vi "io_query_with_OPC_synchro.vi"(7 "Timeout in (0 = OPC timeout)":u32, 8 "error in":errorcluster, 9 "bytes to read (Read all available)":u32, 10 "write buffer":string, 11 "VISA resource name":refnum<visa-resource-name>) -> (0 "error out":errorcluster, 2 "read buffer":string, 3 "VISA resource name out":refnum<visa-resource-name>)   [LabVIEW 2014, in "rszvl_rsidr_core.lvlib"]
uses:
  rszvl_rsidr_core.lvlib
  type_Attribute.ctl
  type_Attribute_Data_Type.ctl
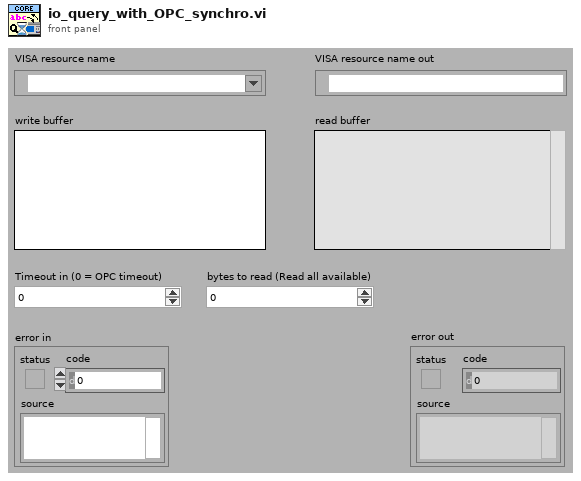
[diagram p1: front panel]
types:
  T1 = typedef "rszvl_rsidr_core.lvlib/type_Session_Data.ctl" = cluster{"Instr type":string, "Instr type for err. msg.":string, "Installed Options":string[], "OPC Timeout":i32, "Query Instrument Status":bool, "Check Range":bool, "Check Options":bool, "Add LF to Write":bool, "Simulate":bool, "Logging":bool, "Logging params":variant, "Interface Type":enum16{"Unknown", "GPIB", "VXI", "GPIB_VXI", "ASRL", "PXI", "TCPIP", "USB", "SOCKET"}, "Fast Sweep":i32, "AdditionalFlags":i32, "WaitBeforeWrite":i32, "WaitBeforeRead":i32, "BinDataChunkSize":i64}
  T2 = enum16{"Unknown", "GPIB", "VXI", "GPIB_VXI", "ASRL", "PXI", "TCPIP", "USB", "SOCKET"}
  T3 = typedef "rszvl_rsidr_core.lvlib/type_Attribute.ctl" = cluster{"Identifier":string, "Descriptive name":string, "Data Type":T4, "Command":string, "Access":u16, "Range Table":string, "Read Callback":string, "Write Callback":string, "Range Callback":string, "Check Callback":string, "Rngtable Callback":string, "Coerce Callback":string, "Supported Models":string, "Instrument Options":string, "Repeated Capabilities":string, "Check Status Callback":string, "Index":i32, "Flag: OPC Wait":bool, "Flag: Dont check status":bool, "Flag: Cache Only":bool}
  T4 = typedef "rszvl_rsidr_core.lvlib/type_Attribute_Data_Type.ctl" = enum16{"Integer 32", "Double", "String", "Boolean", "None", "Integer 64"}
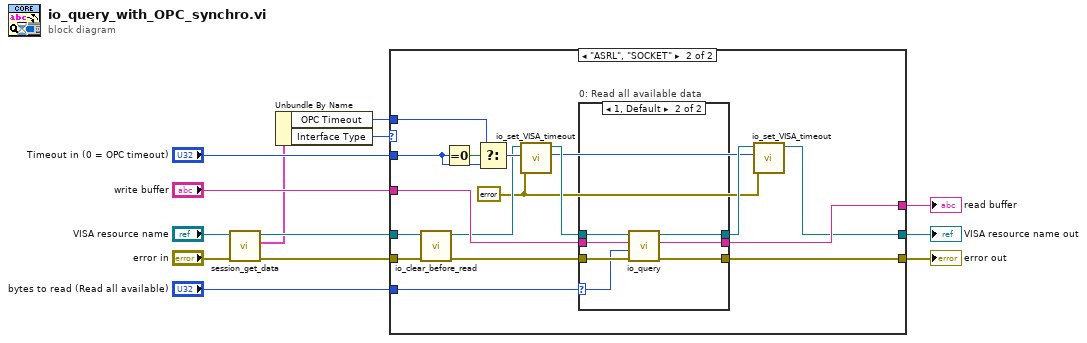
[diagram p0: block diagram]
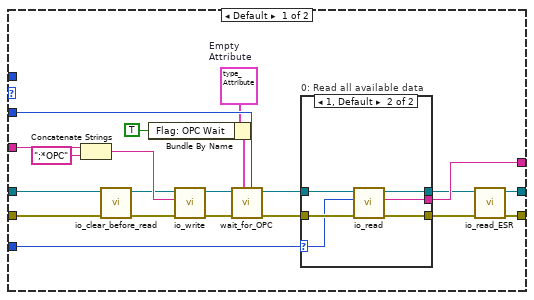
[diagram p2: hidden frame]
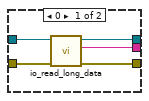
[diagram p3: hidden frame]
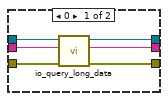
[diagram p4: hidden frame]
diagram:
  n1 = call "session_get_data.vi"("error in"="error in", "VISA resource name"="VISA resource name") -> ("error out"=w5:errorcluster, "Session User Data out"=w2:T1, "VISA resource name out"=w4:refnum<visa-resource-name>)  [unwired: 7 in]
  n2 = Unbundle By Name(w2) -> ("OPC Timeout"=w1:i32, "Interface Type"=w3:T2)
  n3 = case shown="\"ASRL\", \"SOCKET\"" w3 {
    tunnel: "Timeout in (0 = OPC timeout)" -> [w34 w53]
    tunnel: "write buffer" -> [w33 w57]
    tunnel: [w32 w62] -> w11
    tunnel: "bytes to read (Read all available)" -> [w31 w61]
    tunnel: [w30 w58] -> w9
    tunnel: [w29 w48] -> w8
    tunnel: w5 -> [w15 w60]
    tunnel: w4 -> [w14 w59]
    tunnel: w1 -> [_ w52]
    frame Default {
      w20 = T3 {"Identifier"="", "Descriptive name"="", "Data Type"=enum."Integer 32", "Command"="", "Access"=2, "Range Table"="", "Read Callback"="", "Write Callback"="", "Range Callback"="", "Check Callback"="", "Rngtable Callback"="", "Coerce Callback"="", "Supported Models"="", "Instrument Options"="", "Repeated Capabilities"="", "Check Status Callback"="", "Index"=0, "Flag: OPC Wait"=FALSE, "Flag: Dont check status"=FALSE, "Flag: Cache Only"=FALSE}  # Empty Attribute
      n4 = Concatenate Strings(w33, ";*OPC" ("string")) -> (w28:string)
      n5 = call "io_clear_before_read.vi"("error in"=w15, "VISA resource name"=w14) -> ("error out"=w26:errorcluster, "VISA resource name out"=w25:refnum<visa-resource-name>)  [unwired: 8 in]
      n6 = Bundle By Name(cluster=w20, "Flag: OPC Wait"=TRUE) -> (w19:T3)
      n7 = call "io_write.vi"("error in"=w26, "write buffer"=w28, "VISA resource name"=w25) -> ("error out"=w24:errorcluster, "VISA resource name out"=w23:refnum<visa-resource-name>)  [unwired: 7 in]
      n8 = call "wait_for_OPC.vi"("Timeout in (0 = OPC timeout)"=w34, "Attribute"=w19, "error in"=w24, "VISA resource name"=w23) -> ("error out"=w22:errorcluster, "VISA resource name out"=w21:refnum<visa-resource-name>)  [unwired: 6 in]
      n9 = case "0: Read all available data" shown="1, Default" w31 {
        selector: w31 -> [_ w41]
        tunnel: w22 -> [w39 w45]
        tunnel: w21 -> [w38 w44]
        tunnel: [w37 w43] -> w17
        tunnel: [w36 w42] -> w16
        tunnel: [w35 w40] -> w32
        frame 0 {
          n10 = call "io_read_long_data.vi"("error in"=w39, "VISA resource name"=w38) -> ("error out"=w37:errorcluster, "read buffer"=w35:string, "VISA resource name out"=w36:refnum<visa-resource-name>)  [unwired: 6 in, 1 out]
        }
        frame 1, Default {
          n11 = call "io_read.vi"("error in"=w45, "byte count (2048)"=w41, "VISA resource name"=w44) -> ("error out"=w43:errorcluster, "read buffer"=w40:string, "VISA resource name out"=w42:refnum<visa-resource-name>)  [unwired: 5 in, 1 out]
        }
      }
      n12 = call "io_read_ESR.vi"("error in"=w17, "VISA resource name"=w16) -> ("error out"=w30:errorcluster, "VISA resource name out"=w29:refnum<visa-resource-name>)  [unwired: 7 in, 1 out]
    }
    frame "ASRL", "SOCKET" {
      w47 = errorcluster {"status"=FALSE, "code"=0, "source"=""} ("error in")
      n13 = call "io_clear_before_read.vi"("error in"=w60, "VISA resource name"=w59) -> ("error out"=w56:errorcluster, "VISA resource name out"=w51:refnum<visa-resource-name>)  [unwired: 8 in]
      n14 = Equal To 0?(x=w53) -> (x = 0?=w54:bool)
      n15 = Select(t=w52, s=w54, f=w53) -> (s? t:f=w55:u32)
      n16 = call "io_set_VISA_timeout.vi"("error in"=w47, "VISA Timeout"=w55, "VISA resource name"=w51) -> ("Old VISA Timeout"=w46:u32, "VISA resource name out"=w50:refnum<visa-resource-name>)  [unwired: 6 in, 1 out]
      n17 = case "0: Read all available data" shown="1, Default" w61 {
        selector: w61 -> [_ w71]
        tunnel: w56 -> [w68 w75]
        tunnel: w50 -> [w67 w74]
        tunnel: [w66 w73] -> w58
        tunnel: [w65 w72] -> w49
        tunnel: [w64 w70] -> w62
        tunnel: w57 -> [w63 w69]
        frame 0 {
          n18 = call "io_query_long_data.vi"("error in"=w68, "write buffer"=w63, "VISA resource name"=w67) -> ("error out"=w66:errorcluster, "read buffer"=w64:string, "VISA resource name out"=w65:refnum<visa-resource-name>)  [unwired: 6 in]
        }
        frame 1, Default {
          n19 = call "io_query.vi"("error in"=w75, "Bytes to read (2048)"=w71, "write buffer"=w69, "VISA resource name"=w74) -> ("error out"=w73:errorcluster, "read buffer"=w70:string, "VISA resource name out"=w72:refnum<visa-resource-name>)  [unwired: 4 in, 1 out]
        }
      }
      n20 = call "io_set_VISA_timeout.vi"("error in"=w47, "VISA Timeout"=w46, "VISA resource name"=w49) -> ("VISA resource name out"=w48:refnum<visa-resource-name>)  [unwired: 6 in, 2 out]
    }
  }
  "VISA resource name out" <- w8
  "error out" <- w9
  "read buffer" <- w11
